vi "Close.vi"(8 "error in (no error)":errorcluster, 11 "OBS in":refnum<class "OBS.lvclass">) -> (0 "error out":errorcluster, 3 "OBS out":refnum<class "OBS.lvclass">)   [LabVIEW 2022 SP3, in "obs-websocket-lv.lvlib" / "OBS.lvclass"]
uses:
  OBS.lvclass
  OBS.lvclass/OBS.ctl
  Command.ctl
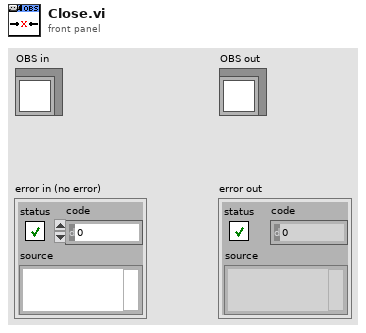
[diagram p1: front panel]
types:
  T1 = typedef "obs-websocket-lv.lvlib/OBS.lvclass/Command.ctl" = enum16{"Open", "Close", "Stop"}
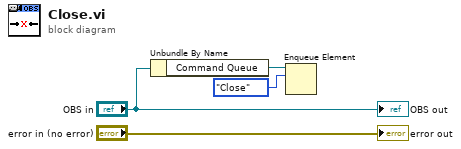
[diagram p0: block diagram]
diagram:
  n1 = Unbundle By Name("OBS in") -> ("Command Queue"=w2:refnum<queue>)
  n2 = Enqueue Element(queue=w2, element=Command."Close") -> ()  [unwired: 2 in, 3 out]
  "error out" <- "error in (no error)"
  "OBS out" <- "OBS in"
